vi "dospi_14052019_grises.vi"() -> (0 "dt (ms) 2":u16=5, 1 "Canal 2":string="X", 2 "InterfaceName":string="cam0", 3 "Puerto 2":refnum<visa-resource-name>="COM2", 4 "Selección Rectángulo (px) 2":T1={"Left"=80, "Top"=180, "Right"=730, "Bottom"=830}, 5 "V 2Pi\nActual":sgl=3.4309938 format="%#.1g")   [LabVIEW 2020]
uses:
  <vilib>/Instr/_visa.llb/VISA Find Search Mode.ctl
  <vilib>/Instr/_visa.llb/VISA Configure Serial Port (Instr).vi
  <vilib>/vision/NI_Vision_Development_Module.lvlib
  <vilib>/gmath/NI_Gmath.lvlib
  <vilib>/vision/driver/NI_Vision_Acquisition_Software.lvlib
  <vilib>/Analysis/NI_AALPro.lvlib
panel:
  in  "Sust":bool=TRUE
  in  "Sustracción 2":bool
  in  "V 2Pi\nApriori":sgl=4.0 min=0.1 max=15 step=0.1 format="%.1f"
  in  "Puerto":refnum<visa-resource-name>="COM2"
  in  "Selección Rectángulo (px)":T1={"Left"=80, "Top"=180, "Right"=730, "Bottom"=830}
  in  "dV (V)":sgl=0.4 min=0.1 max=5 step=0.1 format="%.1f"
  in  "dt (ms)":u16=5
  in  "Rango (V)":u8=7 max=100 step=1
  in  "Canal":string="X"
  out "valor enviado":string="17.2"
  in  "Sustracción":bool
  out "Captura":T2(plugin-control)
  in  "error in (no error)":errorcluster
  out "tiempo total":u32=1016
  out "Ciclos 2Pi":cluster{"xi used":dbl[], "yi":dbl[]}[](graph)=[{"xi used"=[0.0, 0.4000000059604645, 0.800000011920929, 1.2000000476837158, 1.600000023841858, 2.0, 2.4000000953674316, 2.799999952316284, 3.200000047683716, 3.6000001430511475, 4.0, 4.400000095367432, 4.800000190734863, 5.200000286102295, 5.599999904632568, 6.0, 6.400000095367432, 6.800000190734863, 7.200000286102295], "yi"=[1.6194082498550415, 2.081223726272583, 3.9639101028442383, 5.417988300323486, 5.994996547698975, 5.763517379760742, 4.927460193634033, 3.268064022064209, 1.9228070974349976, 2.006049633026123, 3.322584629058838, 5.178757190704346, 5.874281883239746, 5.9817633628845215, 5.3586106300354, 3.7743194103240967, 2.4187028408050537, 2.3153183460235596, 3.7917206287384033]}, {"xi used"=[0.0, 0.10000000149011612, 0.20000000298023224, 0.30000000447034836, 0.4000000059604645, 0.5000000074505806, 0.6000000089406967, 0.7000000104308128, 0.800000011920929, 0.9000000208616257, 1.0000000298023224, 1.100000038743019, 1.2000000476837158, 1.3000000417232513, 1.4000000357627869, 1.5000000298023224, 1.600000023841858, 1.7000000178813934, 1.800000011920929, 1.9000000059604645, 2.0, 2.100000023841858, 2.200000047683716, 2.3000000715255737, 2.4000000953674316, 2.5000000596046448, 2.600000023841858, 2.699999988079071, 2.799999952316284, 2.899999976158142, 3.0, 3.100000023841858, 3.200000047683716, 3.3000000715255737, 3.4000000953674316, 3.5000001192092896, 3.6000001430511475, 3.7000001072883606, 3.8000000715255737, 3.900000035762787, 4.0, 4.100000023841858, 4.200000047683716, 4.300000071525574, 4.400000095367432, 4.5000001192092896, 4.6000001430511475, 4.700000166893005, 4.800000190734863, 4.900000214576721, 5.000000238418579, 5.100000262260437, 5.200000286102295, 5.300000190734863, 5.400000095367432, 5.5, 5.599999904632568, 5.699999928474426, 5.799999952316284, 5.899999976158142, 6.0, 6.100000023841858, 6.200000047683716, 6.300000071525574, 6.400000095367432, 6.5000001192092896, 6.6000001430511475, 6.700000166893005, 6.800000190734863, 6.900000214576721, 7.000000238418579, 7.100000262260437, 7.200000286102295], "yi"=[1.6194082498550415, 1.6415202646400873, 1.700969021152869, 1.835091261121122, 2.081223726272583, 2.4615675244221595, 2.9377812277334487, 3.4563877744572187, 3.9639101028442383, 4.416314498578613, 4.807340439884618, 5.1401707620402455, 5.417988300323486, 5.643229129866736, 5.815342479071086, 5.9330308007455095, 5.994996547698975, 6.0015645873541725, 5.959549445588673, 5.8773880628937665, 5.763517379760742, 5.622745854472534, 5.4453682711596425, 5.218050945615625, 4.927460193634033, 4.566549653810085, 4.153420905030226, 3.7124627576598135, 3.268064022064209, 2.8442846434260165, 2.4638706226251452, 2.1492390703865025, 1.9228070974349976, 1.8016579460584699, 1.7815393847964844, 1.8528653137515367, 2.006049633026123, 2.2327082258196134, 2.529265762805696, 2.8933489839101707, 3.322584629058838, 3.807336769827714, 4.308917005977046, 4.78137419407865, 5.178757190704346, 5.467236063197128, 5.661465721984701, 5.788222288265946, 5.874281883239746, 5.940712665430707, 5.985750942666336, 6.001925060099863, 5.9817633628845215, 5.9173299887642, 5.798831744986865, 5.616011126946077, 5.3586106300354, 5.0225638976458455, 4.628571701943094, 4.203526165358669, 3.7743194103240967, 3.3657338746848104, 2.994113257941885, 2.673691575010305, 2.4187028408050537, 2.2430304554985607, 2.1591553602930404, 2.1792078816481535, 2.3153183460235596, 2.5722541809073114, 2.925331217901028, 3.3425023896347215, 3.7917206287384033]}, {"xi used"=[1.6635191881348852, 5.094512955533968], "yi"=[6.004797437208987, 6.001979760925586]}]
  out "error out":errorcluster
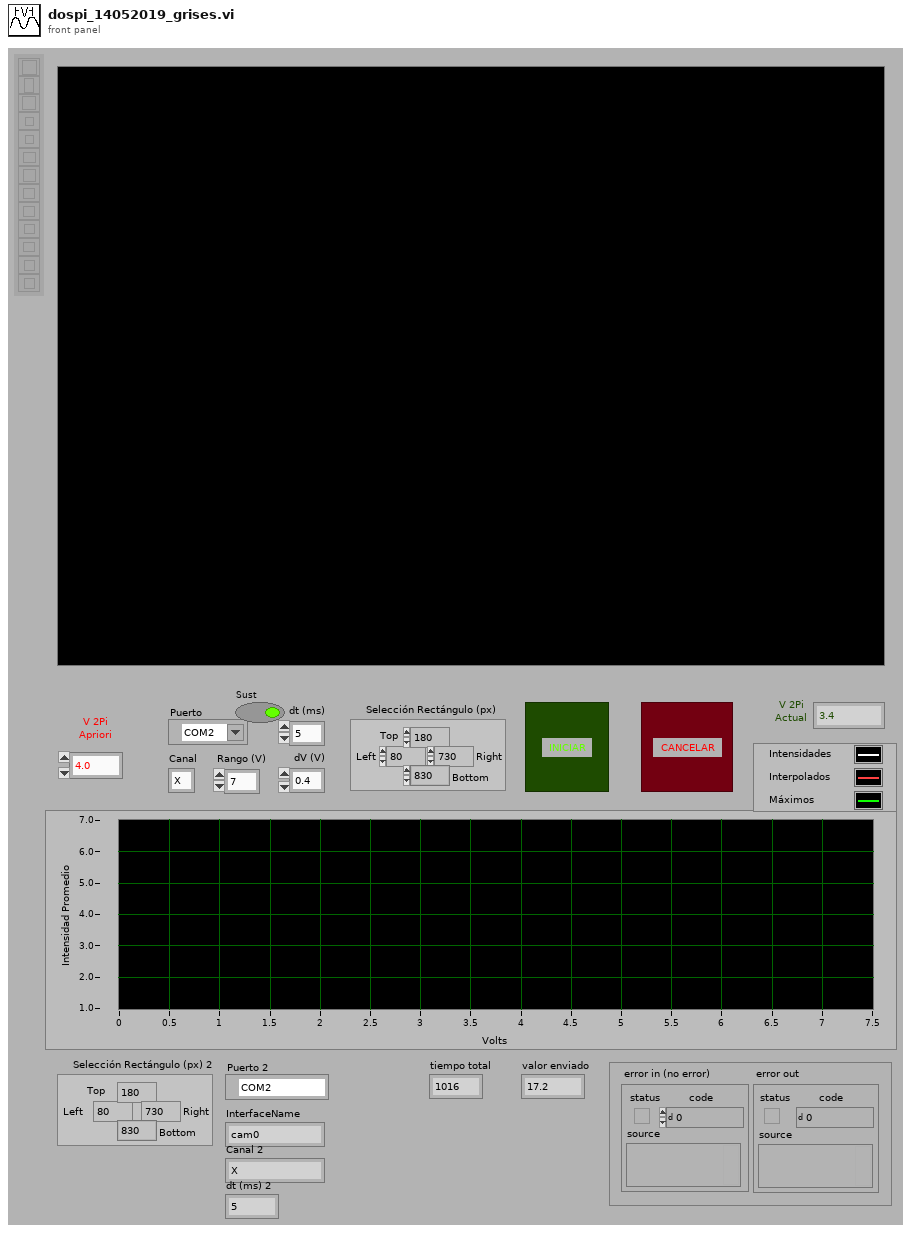
[diagram p1: front panel]
types:
  T1 = cluster{"Left":i32, "Top":i32, "Right":i32, "Bottom":i32}
  T2 = typedef "IMAQ Image.ctl" = refnum<image>
  T3 = typedef "VISA Find Search Mode.ctl" = u32
  T4 = cluster{"Type":u32, "Version":u32, "Flags":u32, "SerialNumberHigh":u32, "SerialNumberLow":u32, "BusType":u32, "InterfaceName":string, "VendorName":string, "ModelName":string, "CameraFileName":string, "CameraAttributeURL":string}[]
  T5 = cluster{"Type":u32, "Version":u32, "Flags":u32, "SerialNumberHigh":u32, "SerialNumberLow":u32, "BusType":u32, "InterfaceName":string, "VendorName":string, "ModelName":string, "CameraFileName":string, "CameraAttributeURL":string}
  T6 = typedef "IMAQdx.ctl" = refnum<k21>
  T7 = cluster{"Mean Value":sgl, "Standard Variation":sgl, "Minimal Value":sgl, "Maximal Value":sgl, "Area (calibrated)":sgl, "Area (pixels)":i32, "%":sgl}
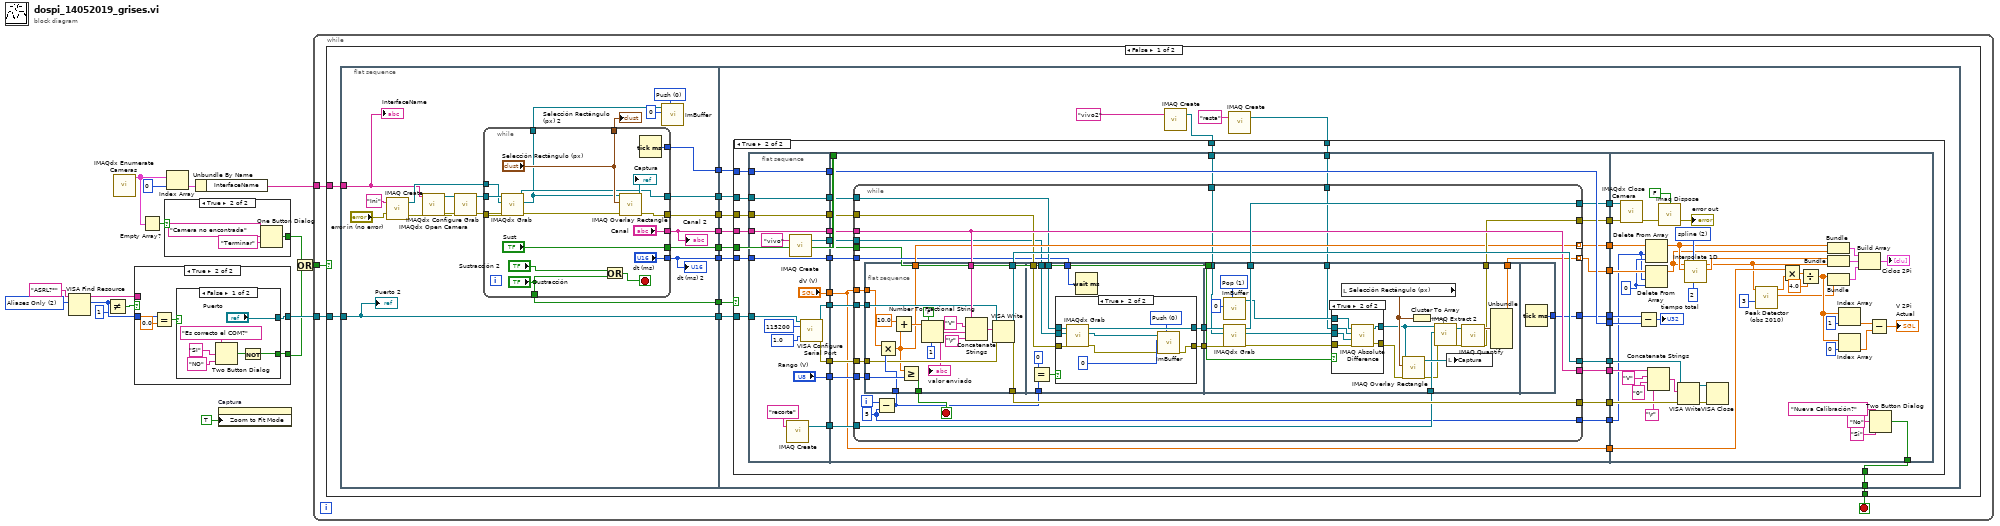
[diagram p0: block diagram]
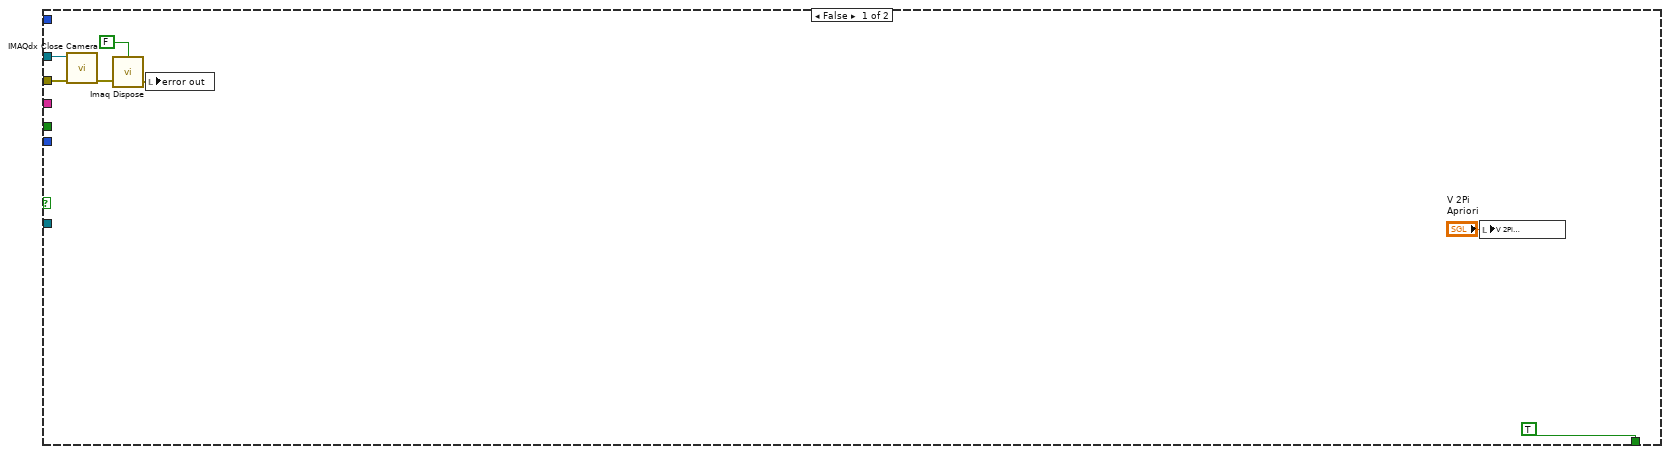
[diagram p2: hidden frame]
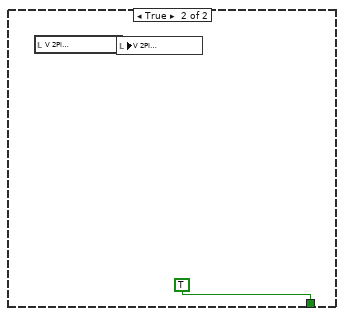
[diagram p5: hidden frame]
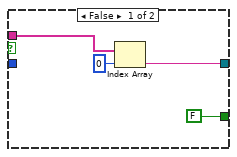
[diagram p6: hidden frame]
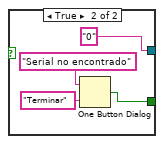
[diagram p7: hidden frame]
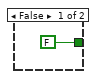
[diagram p8: hidden frame]
diagram:
  w11 = T3 2 items=["Canonical Names Only"=0, "Aliases Only"=2, "Include Matching Aliases"=3, "Include All Aliases"=4] ("Search Mode")
  n1 = VISA Find Resource(10:w11, 11:"ASRL?*" ("expression (\"?*\")")) -> (2:w16:u32, 3:w15:string[])  [unwired: 1 in, 1 out]
  n2 = Not Equal?(x=w16, y=u32 1) -> (x != y?=w14:bool)
  n3 = call <vilib>:"IMAQdx Enumerate Cameras.vi"() -> ("Camera Information Array"=w9:T4)  [unwired: 10 in, 1 out]
  n4 = case shown="True" w14 {
    tunnel: w15 -> [w20 _]
    tunnel: [w18 w25] -> w5
    tunnel: w16 -> [_ w23]
    tunnel: [FALSE ("true") w21] -> w3
    frame False {
      n5 = Index Array(array=w20, index=0) -> (element=w18:string)
    }
    frame True {
      n6 = Equal?(x=w23, y=0.0) -> (x = y?=w22:bool)
      n7 = case shown="False" w22 {
        tunnel: ["Puerto" "0" ("button name (\"OK\")")] -> w25
        tunnel: [w26 w32] -> w21
        frame False {
          n8 = Two Button Dialog(message="Es correcto el COM?" ("error source (\" \")"), 1:"NO" ("F button name (\"Cancel\")"), 2:"SI" ("T button name (\"OK\")")) -> (T button?=w27:bool)
          n9 = Not(x=w27) -> (.not. x?=w26:bool)
        }
        frame True {
          n10 = One Button Dialog(message="Serial no encontrado" ("error source (\" \")"), button name ("OK")="Terminar") -> (true=w32:bool)
        }
      }
    }
  }
  n11 = Empty Array?(array=w9) -> (empty?=w10:bool)
  n12 = case shown="True" w10 {
    tunnel: [FALSE ("true") w37] -> w4
    frame False {
    }
    frame True {
      n13 = One Button Dialog(message="Camera no encontrada" ("error source (\" \")"), button name ("OK")="Terminar") -> (true=w37:bool)
    }
  }
  n14 = Index Array(array=w9, index=0) -> (element=w8:T5)
  n15 = Unbundle By Name(w8) -> ("InterfaceName"=w6:string)
  n16 = property on="Captura" class="ImageControl"("Zoom to Fit Mode"=TRUE) -> ()  [unwired: 2 in, 2 out]
  n17 = Or(x=w4, y=w3) -> (x .or. y?=w2:bool)
  n18 = while {
    tunnel: w6 -> [w43]
    tunnel: w5 -> [w42]
    tunnel: w2 -> [w41]
    stop <- w40 stop-if-true
    n19 = case shown="False" w41 {
      tunnel: w43 -> [w54 _]
      tunnel: w42 -> [w53 _]
      tunnel: [w45 TRUE ("T button?")] -> w40
      frame False {
        n20 = flat-sequence {
          tunnel: w54 -> [w67]
          tunnel: w53 -> [w60]
          tunnel: [w60] -> w52
          tunnel: [w66] -> w51
          tunnel: [w65] -> w50
          tunnel: [w64] -> w49
          tunnel: [w63] -> w48
          tunnel: [w62] -> w47
          tunnel: [w61] -> w46
          tunnel: [w55] -> w44
          tunnel: w52 -> [w104]
          tunnel: w51 -> [w103]
          tunnel: w50 -> [w102]
          tunnel: w49 -> [w101]
          tunnel: w48 -> [w100]
          tunnel: w47 -> [w99]
          tunnel: w46 -> [w98]
          tunnel: [w97] -> w45
          tunnel: w44 -> [w92]
          frame #0 {
            w57 = u16 0 items=["Push", "Pop", "Reset"] ("Function")
            n21 = call "IMAQ Create"("Image Name"="Ini", "error in (no error)"="error in (no error)") -> ("New Image"=w71:T2, "error out"=w68:errorcluster)  [unwired: 3 in]
            n22 = call <vilib>:"IMAQdx Open Camera.vi"("error in"=w68, "Session In"=w67) -> ("error out"=w69:errorcluster, "Session Out"=w70:T6)  [unwired: 8 in]
            n23 = call <vilib>:"IMAQdx Configure Grab.vi"("error in"=w69, "Session In"=w70) -> ("error out"=w72:errorcluster, "Session Out"=w73:T6)  [unwired: 8 in]
            n24 = while {
              tunnel: w72 -> [w90]
              tunnel: [w79] -> w65
              tunnel: w73 -> [w91]
              tunnel: w71 -> [w89]
              tunnel: [w88] -> w66
              tunnel: [w81] -> w64
              tunnel: ["Sustracción"] -> w63
              tunnel: ["Canal"] -> w62
              tunnel: ["dt (ms)"] -> w61
              tunnel: [w77] -> w58
              tunnel: ["Selección Rectángulo (px)"] -> w59
              tunnel: ["Sust"] -> w55
              stop <- w87 stop-if-true
              n25 = call <vilib>:"IMAQdx Grab.vi"("error in"=w90, "Image In"=w89, "Session In"=w91) -> ("error out"=w76:errorcluster, "Image Out"=w77:T2, "Session Out"=w79:T6)  [unwired: 5 in, 1 out]
              n26 = Or(x="Sustracción 2", y="Sustracción") -> (x .or. y?=w87:bool)
              n27 = call "IMAQ Overlay Rectangle"("error in (no error)"=w76, "Rectangle"="Selección Rectángulo (px)", "Image"=w77) -> ("error out"=w81:errorcluster, "Image Out"=→"Captura":T2)  [unwired: 7 in]
              n28 = Tick Count (ms)() -> (millisecond timer value=w88:u32)
            }
            "Canal 2" <- w62
            "dt (ms) 2" <- w61
            "Selección Rectángulo (px) 2" <- w59
            n29 = call "ImBuffer.vi"("Function"=w57, "Buffer #"=0, "Image In"=w58) -> ()  [unwired: 6 in, 3 out]
            "Puerto 2" <- w60
            "InterfaceName" <- w67
          }
          frame #1 {
            n30 = call "IMAQ Create"("Image Name"="vivo2") -> ("New Image"=w93:T2)  [unwired: 4 in, 1 out]
            n31 = call "IMAQ Create"("Image Name"="resta") -> ("New Image"=w95:T2)  [unwired: 4 in, 1 out]
            n32 = case shown="True" w100 {
              tunnel: w104 -> [_ w122]
              tunnel: w103 -> [_ w121]
              tunnel: w102 -> [w111 w120]
              tunnel: w101 -> [w110 w119]
              tunnel: w99 -> [_ w118]
              tunnel: w98 -> [_ w116]
              tunnel: [TRUE ("T button?") w115] -> w97
              tunnel: w95 -> [_ w114]
              tunnel: w93 -> [_ w113]
              tunnel: w92 -> [_ w112]
              frame False {
                n33 = call <vilib>:"IMAQdx Close Camera.vi"("error in"=w110, "Session In"=w111) -> ("error out"=w107:errorcluster)  [unwired: 9 in]
                n34 = call "Imaq Dispose"("All Images? (No)"=FALSE, "error in (no error)"=w107) -> ("error out"=w105:errorcluster)  [unwired: 4 in]
                n35 = local write "error out"(w105) -> ()
                n36 = local write "V 2Pi\nActual"("V 2Pi\nApriori") -> ()
              }
              frame True {
                n37 = flat-sequence {
                  tunnel: ["Rango (V)"] -> w143
                  tunnel: [w144] -> w142
                  tunnel: [w149] -> w141
                  tunnel: [w148] -> w140
                  tunnel: [w150] -> w139
                  tunnel: [w152] -> w138
                  tunnel: [w147] -> w137
                  tunnel: [w155] -> w136
                  tunnel: [w154] -> w135
                  tunnel: ["dV (V)"] -> w134
                  tunnel: w122 -> [w151]
                  tunnel: w121 -> [w150]
                  tunnel: w120 -> [w149]
                  tunnel: w119 -> [w148]
                  tunnel: w118 -> [w147]
                  tunnel: [w146] -> w117
                  tunnel: w116 -> [w146]
                  tunnel: w143 -> [w165]
                  tunnel: w142 -> [w181]
                  tunnel: w141 -> [w182]
                  tunnel: w140 -> [w180]
                  tunnel: w139 -> [w179]
                  tunnel: [w179] -> w133
                  tunnel: [w178] -> w132
                  tunnel: [w177] -> w131
                  tunnel: [w176] -> w130
                  tunnel: [w175] -> w129
                  tunnel: [w174] -> w128
                  tunnel: [w173] -> w127
                  tunnel: [w172] -> w126
                  tunnel: [w171] -> w125
                  tunnel: w138 -> [w170]
                  tunnel: w137 -> [w169]
                  tunnel: w136 -> [w167]
                  tunnel: w135 -> [w168]
                  tunnel: [w166] -> w124
                  tunnel: w134 -> [w164]
                  tunnel: [w164] -> w123
                  tunnel: w117 -> [w163]
                  tunnel: w114 -> [w162]
                  tunnel: w113 -> [w161]
                  tunnel: w112 -> [w160]
                  tunnel: w133 -> [w320]
                  tunnel: w132 -> [w324]
                  tunnel: w131 -> [w323]
                  tunnel: w130 -> [w322]
                  tunnel: w129 -> [w321]
                  tunnel: w128 -> [w310]
                  tunnel: w127 -> [w318]
                  tunnel: w126 -> [w319]
                  tunnel: w125 -> [w312]
                  tunnel: w124 -> [w308]
                  tunnel: w123 -> [w305]
                  tunnel: [w290] -> w115
                  frame #0 {
                    w157 = u16 10 items=["1.0"=10, "1.5"=15, "2.0"=20] ("stop bits (10: 1 bit)")
                    n38 = call "IMAQ Create"("Image Name"="recorte") -> ("New Image"=w152:T2)  [unwired: 4 in, 1 out]
                    n39 = call "IMAQ Create"("Image Name"="vivo") -> ("New Image"=w144:T2)  [unwired: 4 in, 1 out]
                    n40 = call-poly "VISA Configure Serial Port"("VISA resource name"=w151, "baud rate (9600)"=u32 115200, "stop bits (10: 1 bit)"=w157) -> ("VISA resource name out"=w154:refnum<visa-resource-name>, "error out"=w155:errorcluster)  [unwired: 11 in]
                  }
                  frame #1 {
                    n41 = while {
                      tunnel: [w199] -> w174 mode=indexing
                      tunnel: [w203] -> w178
                      tunnel: w169 -> [w203]
                      tunnel: [w204] -> w177
                      tunnel: w168 -> [w205]
                      tunnel: w167 -> [w206]
                      tunnel: w165 -> [w207]
                      tunnel: [w208] -> w176
                      tunnel: w180 -> [w189]
                      tunnel: w181 -> [w185]
                      tunnel: w182 -> [w190]
                      tunnel: [w202] -> w175
                      tunnel: [w196] -> w173
                      tunnel: [w201] -> w172
                      tunnel: [w200] -> w171 mode=indexing
                      tunnel: w170 -> [w198]
                      tunnel: [w194] -> w166
                      tunnel: w164 -> [w193]
                      tunnel: w163 -> [w186]
                      tunnel: w162 -> [w192]
                      tunnel: w161 -> [w184]
                      tunnel: w160 -> [w183]
                      i -> [w195]
                      stop <- w197 stop-if-true
                      w194 = 5 ("x")
                      n42 = flat-sequence {
                        tunnel: w205 -> [w213]
                        tunnel: w206 -> [w216]
                        tunnel: [w224] -> w197
                        tunnel: w191 -> [w221]
                        tunnel: w207 -> [w223]
                        tunnel: w203 -> [w215]
                        tunnel: [w209] -> w200
                        tunnel: [w212] -> w204
                        tunnel: [w211] -> w201
                        tunnel: w193 -> [w210]
                        tunnel: w186 -> [w235]
                        tunnel: w191 -> [w233]
                        tunnel: w190 -> [w231]
                        tunnel: w189 -> [w230]
                        tunnel: [w229] -> w188
                        tunnel: [w228] -> w187
                        tunnel: w185 -> [w227]
                        tunnel: [w265] -> w208
                        tunnel: [w264] -> w202
                        tunnel: [w263] -> w199
                        tunnel: w198 -> [w262]
                        tunnel: w192 -> [w252]
                        tunnel: w188 -> [w258]
                        tunnel: w187 -> [w257]
                        tunnel: w184 -> [w254]
                        tunnel: w183 -> [w249]
                        tunnel: [w278] -> w196
                        frame #0 {
                          n43 = Multiply(x=w210, y=w221) -> (x*y=w209:sgl)
                          n44 = Add(x=sgl 10.0, y=w209) -> (x+y=w226:sgl)
                          n45 = Greater Or Equal?(x=w209, y=w223) -> (x >= y?=w224:bool)
                          n46 = Number To Fractional String(use system decimal point (T)=FALSE, number=w226, precision (6)=i16 1) -> (F-format string=w214:string)  [unwired: 1 in]
                          "valor enviado" <- w214
                          n47 = Concatenate Strings(w215, "V" ("Substring"), w214, "\r") -> (w219:string)
                          n48 = VISA Write(VISA resource name=w213, write buffer=w219, error in (no error)=w216) -> (VISA resource name out=w212:refnum<visa-resource-name>, error out=w211:errorcluster)  [unwired: 1 out]
                        }
                        frame #1 {
                          n49 = Equal?(x=u8 0 ("y"), y=w233) -> (x = y?=w234:bool)
                          n50 = case shown="True" w234 {
                            tunnel: w231 -> [w237 w246]
                            tunnel: [w237 w245] -> w228
                            tunnel: w230 -> [w236 w244]
                            tunnel: [w236 w242] -> w229
                            tunnel: w227 -> [_ w240]
                            frame False {
                            }
                            frame True {
                              w241 = u16 0 items=["Push", "Pop", "Reset"] ("Function")
                              n51 = call <vilib>:"IMAQdx Grab.vi"("error in"=w244, "Image In"=w240, "Session In"=w246) -> ("error out"=w239:errorcluster, "Image Out"=w238:T2, "Session Out"=w245:T6)  [unwired: 5 in, 1 out]
                              n52 = call "ImBuffer.vi"("Function"=w241, "error in (no error)"=w239, "Buffer #"=0, "Image In"=w238) -> ("error out"=w242:errorcluster)  [unwired: 5 in, 2 out]
                            }
                          }
                          n53 = Wait (ms)(milliseconds to wait=w235) -> ()  [unwired: 1 out]
                        }
                        frame #2 {
                          w255 = u16 1 items=["Push", "Pop", "Reset"] ("Function")
                          n54 = call "ImBuffer.vi"("Function"=w255, "Buffer #"=0) -> ("Image Out"=w253:T2)  [unwired: 7 in, 2 out]
                          n55 = call <vilib>:"IMAQdx Grab.vi"("error in"=w258, "Image In"=w254, "Session In"=w257) -> ("error out"=w247:errorcluster, "Image Out"=w248:T2, "Session Out"=w265:T6)  [unwired: 5 in, 1 out]
                          n56 = case shown="True" w249 {
                            tunnel: w247 -> [w271 w277]
                            tunnel: w253 -> [_ w276]
                            tunnel: w248 -> [w270 w275]
                            tunnel: w252 -> [_ w274]
                            tunnel: [w271 w273] -> w251
                            tunnel: [w270 w272] -> w250
                            frame False {
                            }
                            frame True {
                              n57 = call "IMAQ Absolute Difference"("Image Src A"=w276, "Image Dst"=w274, "Image Src B"=w275, "error in (no error)"=w277) -> ("Image Dst Out"=w272:T2, "error out"=w273:errorcluster)  [unwired: 3 in]
                            }
                          }
                          n58 = local read "Selección Rectángulo (px)"() -> (w266:T1)
                          n59 = call "IMAQ Overlay Rectangle"("error in (no error)"=w251, "Rectangle"=w266, "Image"=w250) -> ("error out"=w259:errorcluster, "Image Out"=w267:T2)  [unwired: 7 in]
                          n60 = Cluster To Array(cluster=w266) -> (array=w268:i32[])
                          n61 = call "IMAQ Extract 2"("Optional Rectangle"=w268, "error in (no error)"=w259, "Image Dst"=w262, "Image Src"=w250) -> ("error out"=w261:errorcluster, "Image Dst Out"=w260:T2)  [unwired: 6 in]
                          n62 = local write "Captura"(w267) -> ()
                          n63 = call "IMAQ Quantify"("error in (no error)"=w261, "Image"=w260) -> ("error out"=w264:errorcluster, "Global Report"=w269:T7)  [unwired: 1 in, 1 out]
                          n64 = Unbundle(w269) -> ("Mean Value"=w263:sgl)  [unwired: 6 out]
                        }
                        frame #3 {
                          n65 = Tick Count (ms)() -> (millisecond timer value=w278:u32)
                        }
                      }
                      n66 = Subtract(x=w195, y=w194) -> (x-y=w191:i32)
                    }
                  }
                  frame #2 {
                    w309 = 0 ("index")
                    w313 = 2 items=["nearest", "linear", "spline", "cubic Hermite", "Lagrange"] ("method")
                    n67 = call <vilib>:"IMAQdx Close Camera.vi"("error in"=w321, "Session In"=w322) -> ("error out"=w279:errorcluster)  [unwired: 9 in]
                    n68 = Subtract(x=w318, y=w320) -> (x-y=→"tiempo total":u32)
                    n69 = Delete From Array(array=w312, length=w308, index=w309) -> (array with subset deleted=w311:sgl[])  [unwired: 1 out]
                    n70 = Delete From Array(array=w310, length=w308, index=w309) -> (array with subset deleted=w307:sgl[])  [unwired: 1 out]
                    n71 = Concatenate Strings(w324, "V" ("Substring"), "0" ("Substring"), "\r") -> (w301:string)
                    n72 = call "Imaq Dispose"("All Images? (No)"=FALSE, "error in (no error)"=w279) -> ("error out"=→"error out":errorcluster)  [unwired: 4 in]
                    n73 = VISA Write(VISA resource name=w323, write buffer=w301, error in (no error)=w319) -> (VISA resource name out=w299:refnum<visa-resource-name>, error out=w300:errorcluster)  [unwired: 1 out]
                    n74 = call <vilib>:"Interpolate 1D.vi"("ntimes"=2, "method"=w313, "X"=w311, "Y"=w307) -> ("xi used"=w298:dbl[], "yi"=w285:dbl[])  [unwired: 5 in, 1 out]
                    n75 = VISA Close(VISA resource name=w299, error in (no error)=w300) -> ()  [unwired: 1 out]
                    n76 = call <vilib>:"Peak Detector (obs 2010).vi"("width"=3, "X"=w285) -> ("Amplitudes"=w283:dbl[], "Locations"=w284:dbl[])  [unwired: 5 in, 3 out]
                    n77 = Multiply(x=w305, y=w284) -> (x*y=w297:dbl[])
                    n78 = Divide(x=w297, y=sgl 4.0 ("x")) -> (x/y=w293:dbl[])
                    n79 = Bundle(w311, w307) -> (w316:cluster{sgl[], sgl[]})  [unwired: 1 in]
                    n80 = Bundle("xi used"=w298, "yi"=w285) -> (w315:cluster{"xi used":dbl[], "yi":dbl[]})  [unwired: 1 in]
                    n81 = Bundle(w293, "Amplitudes"=w283) -> (w306:cluster{dbl[], "Amplitudes":dbl[]})  [unwired: 1 in]
                    n82 = Index Array(array=w293, index=1) -> (element=w292:dbl)
                    n83 = Index Array(array=w293, index=0) -> (element=w291:dbl)
                    n84 = Build Array(w316, w315, w306) -> (→"Ciclos 2Pi":cluster{"xi used":dbl[], "Amplitudes":dbl[]}[])
                    n85 = Subtract(x=w292, y=w291) -> (x-y=→"V 2Pi\nActual":dbl)
                    n86 = Two Button Dialog(message="Nueva Calibración?", 1:"Si" ("F button name (\"Cancel\")"), 2:"No" ("F button name (\"Cancel\")")) -> (T button?=w290:bool)
                  }
                }
              }
            }
          }
        }
      }
      frame True {
        n87 = local read "V 2Pi\nApriori"() -> (w326:sgl)
        n88 = local write "V 2Pi\nActual"(w326) -> ()
      }
    }
  }
